vi "Teardown.vi"(8 "error in (no error)":errorcluster, 11 "LUnit Mock Class Generator Test In":refnum<class "Pure Mock Class Generator Test.lvclass">) -> (0 "error out":errorcluster, 3 "LUnit Mock Class Generator Test Out":refnum<class "Pure Mock Class Generator Test.lvclass">)   [LabVIEW 2020, in "Pure Mock Class Generator Test.lvclass"]
uses:
  Pure Mock Class Generator Test.lvclass
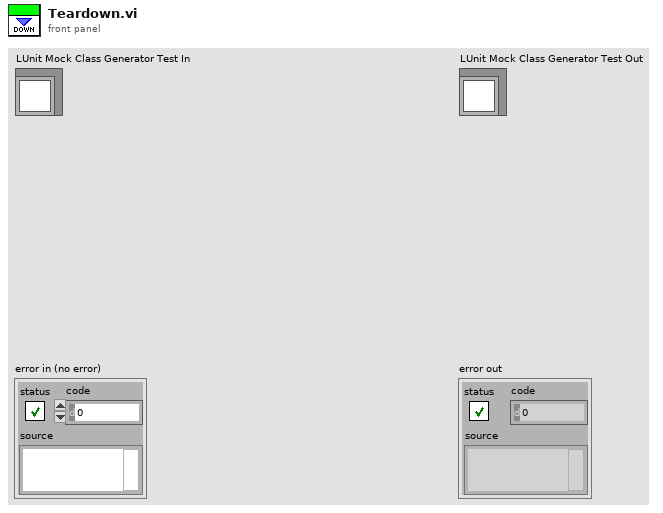
[diagram p1: front panel]
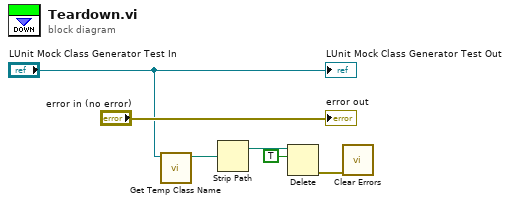
[diagram p0: block diagram]
diagram:
  n1 = call "Get Temp Class Name.vi"("Mock Class Generator Test in"="LUnit Mock Class Generator Test In") -> ("Test Class Path"=w4:path)  [unwired: 10 in]
  n2 = Strip Path(path=w4) -> (stripped path=w2:path)  [unwired: 1 out]
  n3 = Delete(path (use dialog)=w2, entire hierarchy (F)=TRUE) -> (error out=w3:errorcluster)  [unwired: 3 in, 2 out]
  n4 = call <vilib>:"Clear Errors.vi"("error in (no error)"=w3) -> ()  [unwired: 5 in, 2 out]
  "error out" <- "error in (no error)"
  "LUnit Mock Class Generator Test Out" <- "LUnit Mock Class Generator Test In"
